vi "Read Output Folder Path (SubVI).vi"(11 "Settings File Name":path=path "C:/MWT/Config.ini") -> (3 "Output Folder":string)   [LabVIEW 2020]
uses:
  <vilib>/Utility/config.llb/Read Key (String).vi
  <vilib>/Utility/config.llb/Write Key (String).vi
  <vilib>/Utility/config.llb/NI_LVConfig.lvlib
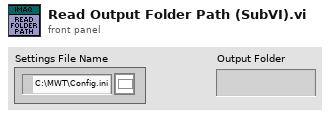
[diagram p1: front panel]
types:
  T1 = typedef "NI_LVConfig.lvlib/Config Data RefNum.ctl" = refnum<k1>
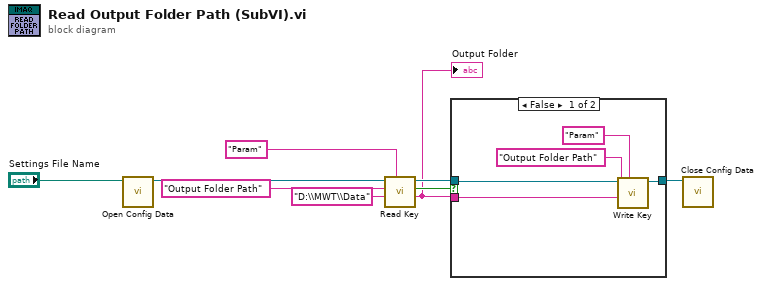
[diagram p0: block diagram]
diagram:
  n1 = call <vilib>:"Open Config Data.vi"("configuration file path"="Settings File Name") -> ("refnum"=w7:T1)  [unwired: 8 in, 2 out]
  n2 = call-poly <vilib>:"Read Key.vi"("section"="Param", "default value"="D:\\MWT\\Data", "key"="Output Folder Path" ("section"), "refnum"=w7) -> ("value"=w2:string, "found?"=w5:bool, "refnum out"=w4:T1)  [unwired: 4 in, 1 out]
  "Output Folder" <- w2
  n3 = case shown="False" w5 {
    tunnel: w4 -> [w12 w15]
    tunnel: [w11 w15] -> w3
    tunnel: w2 -> [w10 _]
    frame False {
      n4 = call-poly <vilib>:"Write Key.vi"("section"="Param", "value"=w10, "key"="Output Folder Path" ("section"), "refnum"=w12) -> ("refnum out"=w11:T1)  [unwired: 5 in, 2 out]
    }
    frame True {
    }
  }
  n5 = call <vilib>:"Close Config Data.vi"("refnum"=w3) -> ()  [unwired: 9 in, 2 out]
